vi "LevyLab Instrument.getAll.vi"(8 "error in (no error)":errorcluster, 11 "ExampleInstrument in":refnum<class "Example.lvclass">) -> (0 "error out":errorcluster, 2 "getAll":T1, 3 "ExampleInstrument out":refnum<class "Example.lvclass">)   [LabVIEW 2019, in "Example.lvclass"]
uses:
  Example.lvclass
  Typedefs/LevyLab Instrument.getAll--Cluster.ctl
  caf7fc02-a1f0-4077-bb00-48bdf0fcd3b8.vi
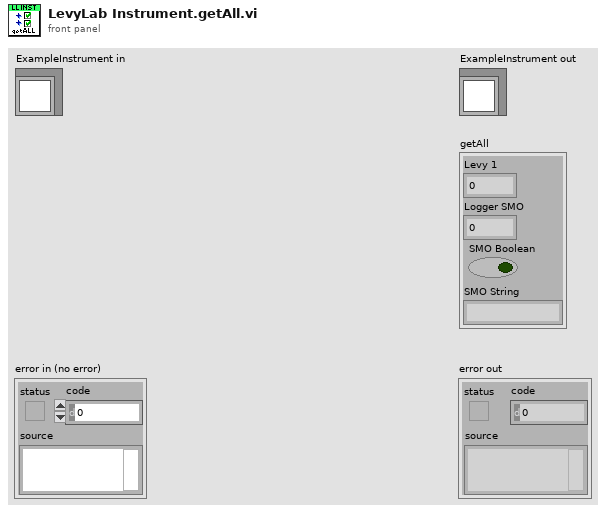
[diagram p1: front panel]
types:
  T1 = typedef "Example.lvclass/LevyLab Instrument.getAll--Cluster.ctl" = cluster{"Levy 1":dbl, "Logger SMO":dbl, "SMO Boolean":bool, "SMO String":string}
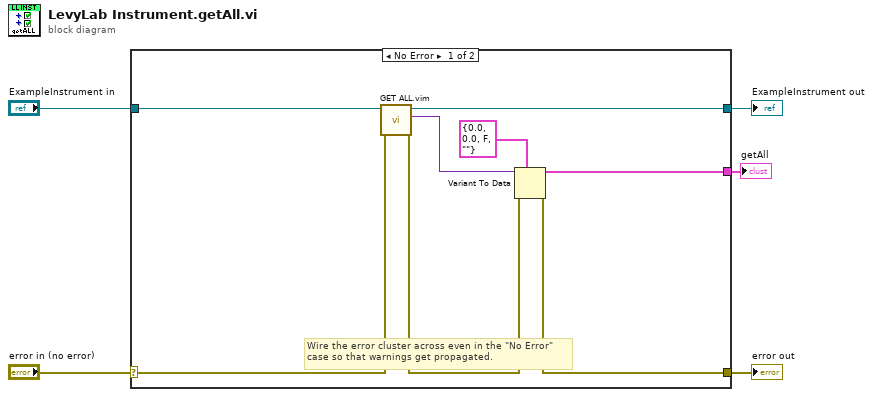
[diagram p0: block diagram]
diagram:
  n1 = case shown="No Error" "error in (no error)" {
    selector: "error in (no error)" -> [w10 w15]
    tunnel: [w8 w15] -> w4
    tunnel: [w11 w14] -> w2
    tunnel: "ExampleInstrument in" -> [w12 w14]
    tunnel: [w7 _] -> w1
    frame No Error {
      # "Wire the error cluster across even in the \"No Error\"\ncase so that warnings get propagated."
      n2 = call "GET ALL.vim"("error in (no error)"=w10, "Instrument in"=w12) -> ("error out"=w9:errorcluster, "getAll"=w6:variant, "Instrument out"=w11:refnum<class "Example.lvclass">)  [unwired: 7 in]
      n3 = Variant To Data(error in=w9, type=T1 {"Levy 1"=0.0, "Logger SMO"=0.0, "SMO Boolean"=FALSE, "SMO String"=""} ("getAll"), Variant=w6) -> (data=w7:T1, error out=w8:errorcluster)
    }
    frame Error {
    }
  }
  "error out" <- w4
  "ExampleInstrument out" <- w2
  "getAll" <- w1
